vi "read_tags_subvi.vi"(2 "USER-T-in":refnum<class "NI Skyline Tag.lvclass">, 3 "STOP-in":refnum<class "NI Skyline Tag.lvclass">) -> (0 "USER-T-out":refnum<class "NI Skyline Tag.lvclass">, 1 "STOP-out":refnum<class "NI Skyline Tag.lvclass">, 4 "StopWeb":bool, 5 "User-T-int":i32)   [LabVIEW 2021]
uses:
  <vilib>/Skyline/Tag/Wrapper/Wrapper_class/NI Skyline Tag.lvclass
  <vilib>/Skyline/Tag/Wrapper/Wrapper_class/Read Tag (I32).vi
  <vilib>/Skyline/Tag/Wrapper/Wrapper_class/Read Tag (Boolean).vi
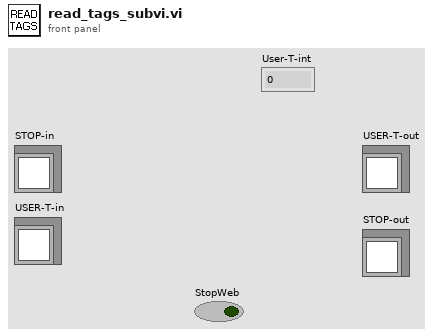
[diagram p1: front panel]
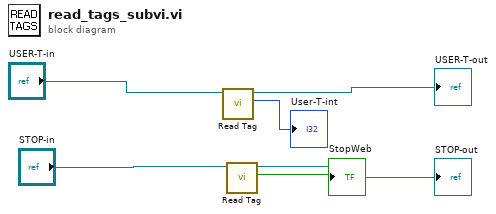
[diagram p0: block diagram]
diagram:
  n1 = call-poly <vilib>:"Read Tag.vi"("tag in"="USER-T-in") -> ("value"=→"User-T-int":i32, "tag out"=→"USER-T-out":refnum<class "NI Skyline Tag.lvclass">)  [unwired: 6 in, 3 out]
  n2 = call-poly <vilib>:"Read Tag.vi"("tag in"="STOP-in") -> ("value"=→"StopWeb":bool, "tag out"=→"STOP-out":refnum<class "NI Skyline Tag.lvclass">)  [unwired: 6 in, 3 out]
